vi "Search Data Folder.vi"(8 "error in (no error)":errorcluster, 11 "Server File List":string[](array[string])) -> (0 "error out":errorcluster, 2 "Disabled Items":i32[](array[numeric]))   [LabVIEW 2019]
doc: "Author: Scott Hannahs <sth@magnet.fsu.edu>\nCopyright 2018 Florida State University, All rights reserved."
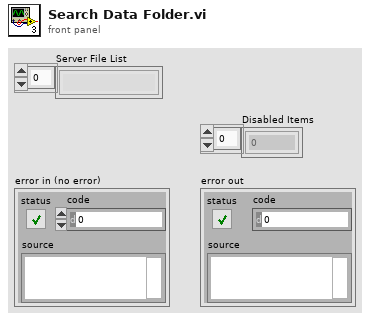
[diagram p1: front panel]
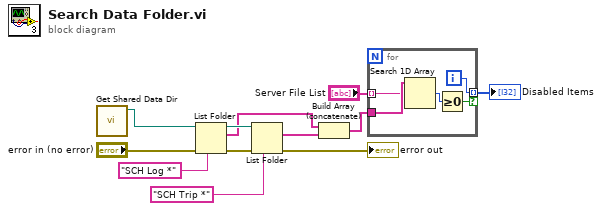
[diagram p0: block diagram]
diagram:
  n1 = call "Get Shared Data Dir.vi"() -> ("Data Directory Path"=w5:path)  [unwired: 2 in, 1 out]
  n2 = List Folder(path=w5, pattern="SCH Log *", error in="error in (no error)") -> (path out=w4:path, filenames=w1:string[], error out=w6:errorcluster)  [unwired: 1 in, 1 out]
  n3 = List Folder(path=w4, pattern="SCH Trip *", error in=w6) -> (filenames=w2:string[], error out=→"error out":errorcluster)  [unwired: 1 in, 2 out]
  n4 = Build Array (concatenate)(w1, w2) -> (w3:string[])
  n5 = for {
    tunnel: w3 -> [w17]
    tunnel: "Server File List" -> [w16] mode=indexing
    tunnel: [w14] -> w10 mode=indexing if=w13
    i -> [w14]
    n6 = Search 1D Array(1D array=w17, element=w16) -> (index of element=w15:i32)  [unwired: 1 in]
    n7 = Greater Or Equal To 0?(x=w15) -> (x >= 0?=w13:bool)
  }
  "Disabled Items" <- w10
